vi "GSP_Manager_Slit_driver.vi"(4 "error in (no error)":errorcluster, 5 "Slit # (Move/Rotate Only)":i32, 6 "Action":T1) -> (0 "error out":errorcluster, 3 "reference out (launch only)":refnum<vi>)   [LabVIEW 2015]
doc: "Provides an interface to the Slit Manager. See the actions below.\n\nLaunch - launch the manager thread supplying references to the controls that the thread will update.\n\nHome - Home the Slit Assembly (translation and rotation motors)\n\nMove - Change to the slit supplied by Slit# (0 == no slit)\n\nShutdown - Shutdown the Slit manager \n\nShow - Move the mask into the beam\n\nHide - Move the mask out of the beam"
uses:
  slitactions.ctl
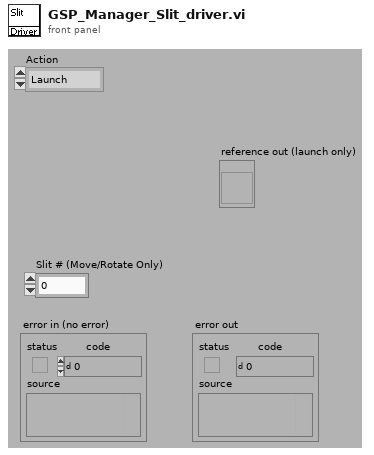
[diagram p1: front panel]
types:
  T1 = typedef "slitactions.ctl" = enum16{"Launch", "INIT_CTL", "Restart", "Show", "Hide", "Home", "Move", "Rotate Only", "Shutdown"}
  T2 = cluster{string, "type string":i16[], "data string":string}
  T3 = cluster{string, "type string":i16[], "data string":string}[]
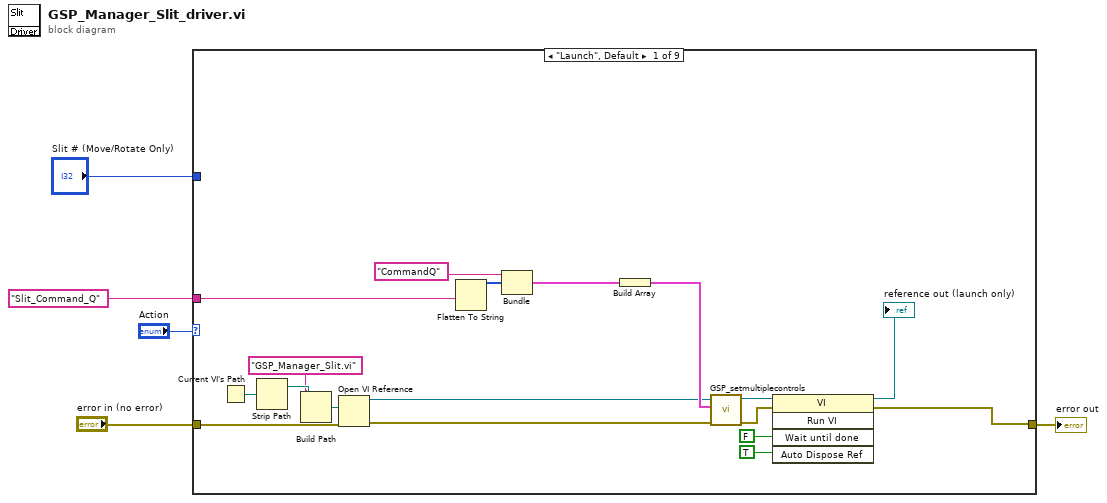
[diagram p0: block diagram]
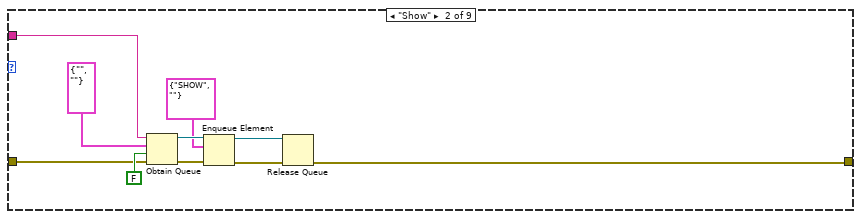
[diagram p2: hidden frame]
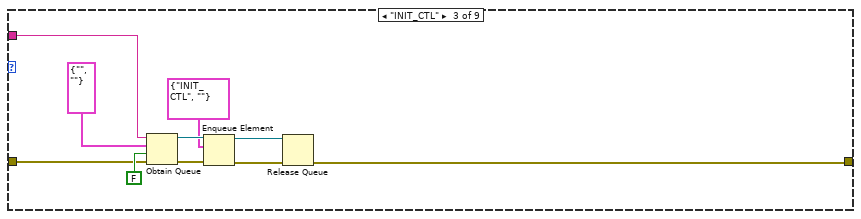
[diagram p3: hidden frame]
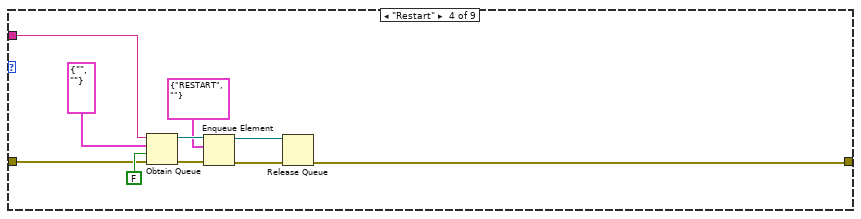
[diagram p4: hidden frame]
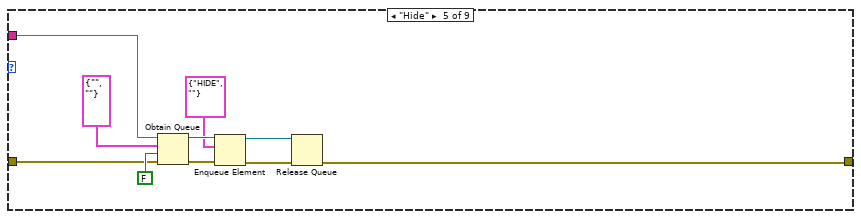
[diagram p5: hidden frame]
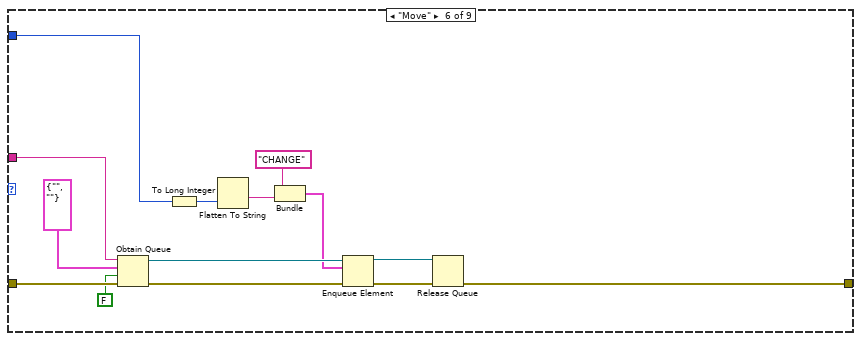
[diagram p6: hidden frame]
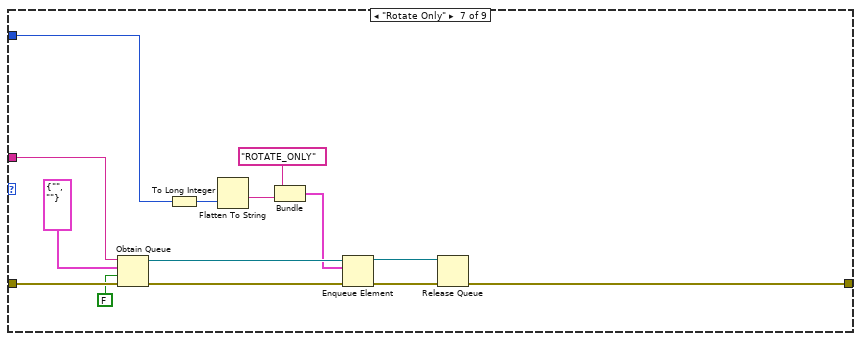
[diagram p7: hidden frame]
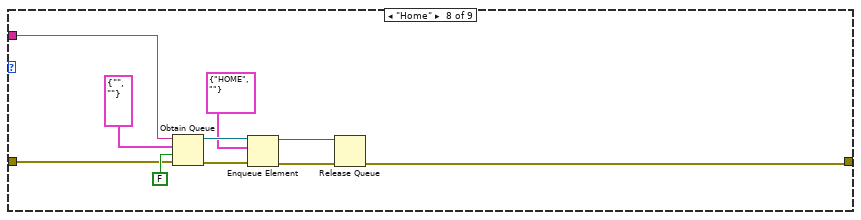
[diagram p8: hidden frame]
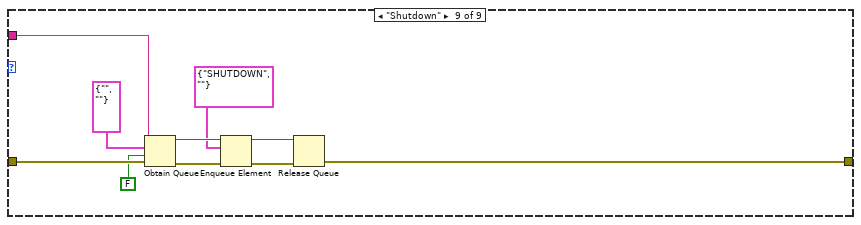
[diagram p9: hidden frame]
diagram:
  n1 = case shown="\"Launch\", Default" "Action" {
    tunnel: "error in (no error)" -> [w19 w31 w41 w51 w61 w78 w92 w99 w112]
    tunnel: [w7 w25 w35 w45 w55 w65 w79 w93 w103] -> w3
    tunnel: "Slit_Command_Q" -> [w8 w30 w40 w50 w60 w77 w91 w98 w110]
    tunnel: "Slit # (Move/Rotate Only)" -> [_ _ _ _ _ w68 w82 _ _]
    frame "Launch", Default {
      n2 = Current VI's Path() -> (path=w12:path)
      n3 = Strip Path(path=w12) -> (stripped path=w10:path)  [unwired: 1 out]
      n4 = Build Path(base path=w10, name or relative path="GSP_Manager_Slit.vi" ("vi path")) -> (appended path=w11:path)
      n5 = Open VI Reference(vi path=w11, error in (no error)=w19) -> (vi reference=w17:refnum<vi>, error out=w18:errorcluster)  [unwired: 4 in]
      n6 = Flatten To String(anything=w8) -> (data string=w22:string, type string=w23:i16[])  [unwired: 3 in, 1 out]
      n7 = Bundle("CommandQ", "type string"=w23, "data string"=w22) -> (w21:T2)  [unwired: 1 in]
      n8 = Build Array(w21) -> (w20:T3)
      n9 = call "GSP_setmultiplecontrols.vi"("error in (no error)"=w18, "Control Infos"=w20, "reference"=w17) -> ("error out"=w15:errorcluster, "reference out"=w16:refnum<vi>)  [unwired: 3 in]
      n10 = invoke class="VI" method="Run VI"(reference=w16, error in=w15, "Wait until done"=FALSE, "Auto Dispose Ref"=TRUE) -> (reference out=→"reference out (launch only)":refnum<vi>, error out=w7:errorcluster)  [unwired: 1 in, 3 out]
    }
    frame "Show" {
      n11 = Obtain Queue(name (unnamed)=w30, element data type=cluster{string, string} {"", ""}, create if not found? (T)=FALSE, error in (no error)=w31) -> (queue out=w34:refnum<queue>, error out=w33:errorcluster)  [unwired: 1 in, 1 out]
      n12 = Enqueue Element(queue=w34, element=cluster{string, string} {"SHOW", ""}, error in (no error)=w33) -> (queue out=w27:refnum<queue>, error out=w26:errorcluster)  [unwired: 1 in, 1 out]
      n13 = Release Queue(queue=w27, error in (no error)=w26) -> (error out=w25:errorcluster)  [unwired: 1 in, 2 out]
    }
    frame "INIT_CTL" {
      n14 = Obtain Queue(name (unnamed)=w40, element data type=cluster{string, string} {"", ""}, create if not found? (T)=FALSE, error in (no error)=w41) -> (queue out=w44:refnum<queue>, error out=w43:errorcluster)  [unwired: 1 in, 1 out]
      n15 = Enqueue Element(queue=w44, element=cluster{string, string} {"INIT_CTL", ""}, error in (no error)=w43) -> (queue out=w37:refnum<queue>, error out=w36:errorcluster)  [unwired: 1 in, 1 out]
      n16 = Release Queue(queue=w37, error in (no error)=w36) -> (error out=w35:errorcluster)  [unwired: 1 in, 2 out]
    }
    frame "Restart" {
      n17 = Obtain Queue(name (unnamed)=w50, element data type=cluster{string, string} {"", ""}, create if not found? (T)=FALSE, error in (no error)=w51) -> (queue out=w54:refnum<queue>, error out=w53:errorcluster)  [unwired: 1 in, 1 out]
      n18 = Enqueue Element(queue=w54, element=cluster{string, string} {"RESTART", ""}, error in (no error)=w53) -> (queue out=w47:refnum<queue>, error out=w46:errorcluster)  [unwired: 1 in, 1 out]
      n19 = Release Queue(queue=w47, error in (no error)=w46) -> (error out=w45:errorcluster)  [unwired: 1 in, 2 out]
    }
    frame "Hide" {
      n20 = Obtain Queue(name (unnamed)=w60, element data type=cluster{string, string} {"", ""}, create if not found? (T)=FALSE, error in (no error)=w61) -> (queue out=w64:refnum<queue>, error out=w63:errorcluster)  [unwired: 1 in, 1 out]
      n21 = Enqueue Element(queue=w64, element=cluster{string, string} {"HIDE", ""}, error in (no error)=w63) -> (queue out=w57:refnum<queue>, error out=w56:errorcluster)  [unwired: 1 in, 1 out]
      n22 = Release Queue(queue=w57, error in (no error)=w56) -> (error out=w55:errorcluster)  [unwired: 1 in, 2 out]
    }
    frame "Move" {
      n23 = Obtain Queue(name (unnamed)=w77, element data type=cluster{string, string} {"", ""}, create if not found? (T)=FALSE, error in (no error)=w78) -> (queue out=w76:refnum<queue>, error out=w75:errorcluster)  [unwired: 1 in, 1 out]
      n24 = To Long Integer(number=w68) -> (32bit integer=w71:i32)
      n25 = Flatten To String(anything=w71) -> (data string=w70:string)  [unwired: 3 in, 2 out]
      n26 = Bundle("CHANGE", "data string"=w70) -> (w72:cluster{string, "data string":string})  [unwired: 1 in]
      n27 = Enqueue Element(queue=w76, element=w72, error in (no error)=w75) -> (queue out=w67:refnum<queue>, error out=w66:errorcluster)  [unwired: 1 in, 1 out]
      n28 = Release Queue(queue=w67, error in (no error)=w66) -> (error out=w65:errorcluster)  [unwired: 1 in, 2 out]
    }
    frame "Rotate Only" {
      n29 = Obtain Queue(name (unnamed)=w91, element data type=cluster{string, string} {"", ""}, create if not found? (T)=FALSE, error in (no error)=w92) -> (queue out=w90:refnum<queue>, error out=w89:errorcluster)  [unwired: 1 in, 1 out]
      n30 = To Long Integer(number=w82) -> (32bit integer=w85:i32)
      n31 = Flatten To String(anything=w85) -> (data string=w84:string)  [unwired: 3 in, 2 out]
      n32 = Bundle("ROTATE_ONLY", "data string"=w84) -> (w86:cluster{string, "data string":string})  [unwired: 1 in]
      n33 = Enqueue Element(queue=w90, element=w86, error in (no error)=w89) -> (queue out=w81:refnum<queue>, error out=w80:errorcluster)  [unwired: 1 in, 1 out]
      n34 = Release Queue(queue=w81, error in (no error)=w80) -> (error out=w79:errorcluster)  [unwired: 1 in, 2 out]
    }
    frame "Home" {
      n35 = Obtain Queue(name (unnamed)=w98, element data type=cluster{string, string} {"", ""}, create if not found? (T)=FALSE, error in (no error)=w99) -> (queue out=w102:refnum<queue>, error out=w101:errorcluster)  [unwired: 1 in, 1 out]
      n36 = Enqueue Element(queue=w102, element=cluster{string, string} {"HOME", ""}, error in (no error)=w101) -> (queue out=w95:refnum<queue>, error out=w94:errorcluster)  [unwired: 1 in, 1 out]
      n37 = Release Queue(queue=w95, error in (no error)=w94) -> (error out=w93:errorcluster)  [unwired: 1 in, 2 out]
    }
    frame "Shutdown" {
      n38 = Obtain Queue(name (unnamed)=w110, element data type=cluster{string, string} {"", ""}, create if not found? (T)=FALSE, error in (no error)=w112) -> (queue out=w109:refnum<queue>, error out=w111:errorcluster)  [unwired: 1 in, 1 out]
      n39 = Enqueue Element(queue=w109, element=cluster{string, string} {"SHUTDOWN", ""}, error in (no error)=w111) -> (queue out=w105:refnum<queue>, error out=w104:errorcluster)  [unwired: 1 in, 1 out]
      n40 = Release Queue(queue=w105, error in (no error)=w104) -> (error out=w103:errorcluster)  [unwired: 1 in, 2 out]
    }
  }
  "error out" <- w3
